vi "Gains fgv.vi"(7 "Mode":T1=enum."Get", 8 "error in (no error)":errorcluster, 10 "Offset":dbl, 11 "Gain":dbl) -> (0 "error out":errorcluster, 2 "Offset":dbl, 3 "Gain":dbl)   [LabVIEW 2016]
uses:
  Controls/Gain modes.ctl
  <vilib>/Utility/file.llb/Read Delimited Spreadsheet (DBL).vi
  <vilib>/Utility/file.llb/Write Delimited Spreadsheet (DBL).vi
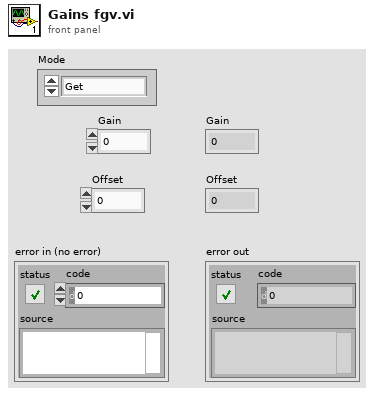
[diagram p1: front panel]
types:
  T1 = typedef "Gain modes.ctl" = enum16{"Initalise", "Get", "Set"}
  T2 = typedef "References.ctl" = cluster{"Tab Control":refnum<vi>, "Logo 1":refnum<vi>, "Logo 2":refnum<vi>, "Connect Actuator":refnum<vi>, "LIVE DATA":refnum<vi>, "Speed":refnum<vi>, "Home position":refnum<vi>, "Limit position":refnum<vi>, "Trigger":refnum<vi>, "Current position":refnum<vi>, "Connect Camera":refnum<vi>, "TEST DATA":refnum<vi>, "LIVE DATA Force":refnum<vi>, "Connect DAQ":refnum<vi>, "Initialised":refnum<vi>, "Test":refnum<vi>}
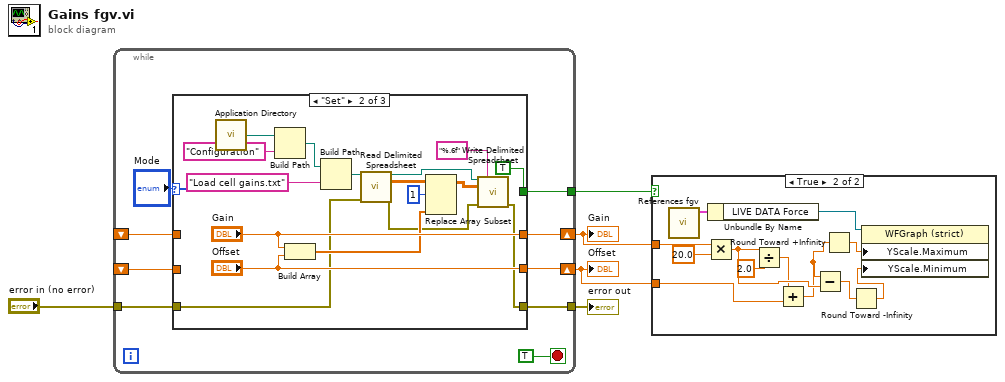
[diagram p0: block diagram]
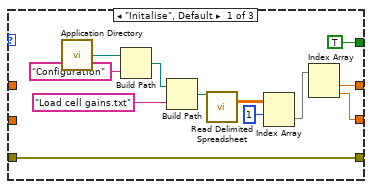
[diagram p3: hidden frame]
diagram:
  n1 = while {
    shift-right: [w10] -> w3
    shift-left: _ -> [w13]
    shift-right: [w11] -> w2
    shift-left: _ -> [w12]
    tunnel: "error in (no error)" -> [w9]
    tunnel: [w8] -> w4
    tunnel: [w6] -> w1
    stop <- TRUE stop-if-true
    n2 = case shown="\"Set\"" "Mode" {
      tunnel: w13 -> [_ _ w46]
      tunnel: w12 -> [_ _ w45]
      tunnel: [w17 "Offset" w45] -> w11
      tunnel: [w18 "Gain" w46] -> w10
      tunnel: w9 -> [w16 w29 w44]
      tunnel: [w16 w28 w44] -> w8
      tunnel: [TRUE TRUE _] -> w6
      frame "Initalise", Default {
        n3 = call <vilib>:"Application Directory.vi"() -> ("Application Directory"=w26:path)
        n4 = Build Path(base path=w26, name or relative path="Configuration") -> (appended path=w24:path)
        n5 = Build Path(base path=w24, name or relative path="Load cell gains.txt") -> (appended path=w22:path)
        n6 = call-poly <vilib>:"Read Delimited Spreadsheet.vi"("file path (dialog if empty)"=w22) -> ("all rows"=w21:dbl[][])  [unwired: 9 in, 5 out]
        n7 = Index Array(array=w21, index (row)=1) -> (element=w19:dbl[])  [unwired: 1 in]
        n8 = Index Array(array=w19) -> (element #1=w18:dbl, element #2=w17:dbl)  [unwired: 2 in]
      }
      frame "Set" {
        n9 = call <vilib>:"Application Directory.vi"() -> ("Application Directory"=w43:path)
        n10 = Build Path(base path=w43, name or relative path="Configuration") -> (appended path=w41:path)
        n11 = Build Array("Gain", "Offset") -> (w34:dbl[])
        n12 = Build Path(base path=w41, name or relative path="Load cell gains.txt") -> (appended path=w39:path)
        n13 = call-poly <vilib>:"Read Delimited Spreadsheet.vi"("file path (dialog if empty)"=w39, "error in (no error)"=w29) -> ("new file path (Not A Path if cancelled)"=w31:path, "all rows"=w38:dbl[][], "error out"=w30:errorcluster)  [unwired: 8 in, 3 out]
        n14 = Replace Array Subset(array=w38, new element=w34, index (row)=1) -> (w32:dbl[][])  [unwired: 1 in]
        n15 = call-poly <vilib>:"Write Delimited Spreadsheet.vi"("file path (dialog if empty)"=w31, "format (%.3f)"="%.6f", "2D data"=w32, "error in (no error)"=w30) -> ("error out"=w28:errorcluster)  [unwired: 10 in, 1 out]
      }
      frame "Get" {
      }
    }
  }
  "Offset" <- w2
  "Gain" <- w3
  "error out" <- w4
  n16 = case shown="True" w1 {
    tunnel: w3 -> [_ w56]
    tunnel: w2 -> [_ w54]
    frame False {
    }
    frame True {
      n17 = call "References fgv.vi"() -> ("Cluster"=w57:T2)  [unwired: 10 in, 1 out]
      n18 = Multiply(x=w56, y=20.0) -> (x*y=w52:dbl)
      n19 = Unbundle By Name(w57) -> ("LIVE DATA Force"=w58:refnum<vi>)
      n20 = Divide(x=w52, y=2.0) -> (x/y=w51:dbl)
      n21 = Add(x=w51, y=w54) -> (x+y=w48:dbl)
      n22 = Subtract(x=w48, y=w52) -> (x-y=w50:dbl)
      n23 = Round Toward +Infinity(x=w48) -> (ceil(x): smallest int >= x=w47:dbl)
      n24 = Round Toward -Infinity(1:w50) -> (0:w49:dbl)
      n25 = property class="WFGraph (strict)"(reference=w58, "YScale.Maximum"=w47, "YScale.Minimum"=w49) -> ()  [unwired: 1 in, 2 out]
    }
  }
